vi "save_scope_config.vi"(0 "Current VI's Path":path=path "" caption="start path", 2 "Save File Type":u16(ring) items=["Automatic Save", "Custom File"], 7 "Controls cluster":T4 {"C1 vertical coupling / V" items=["AC", "DC", "Ground"]; "C2 vertical coupling / V" items=["AC", "DC", "Ground"]; "Trigger slope" items=["Positive", "Negative"]}, 11 "error in":errorcluster) -> (8 "Controls cluster out":T4 {"C1 vertical coupling / V" items=["AC", "DC", "Ground"]; "C2 vertical coupling / V" items=["AC", "DC", "Ground"]; "Trigger slope" items=["Positive", "Negative"]}, 15 "error out":errorcluster)   [LabVIEW 2023]
uses:
  <instrlib>/niScope/Controls/niScope vertical coupling.ctl
  <instrlib>/niScope/Controls/niScope trigger source.ctl
  <instrlib>/niScope/Controls/niScope trigger slope.ctl
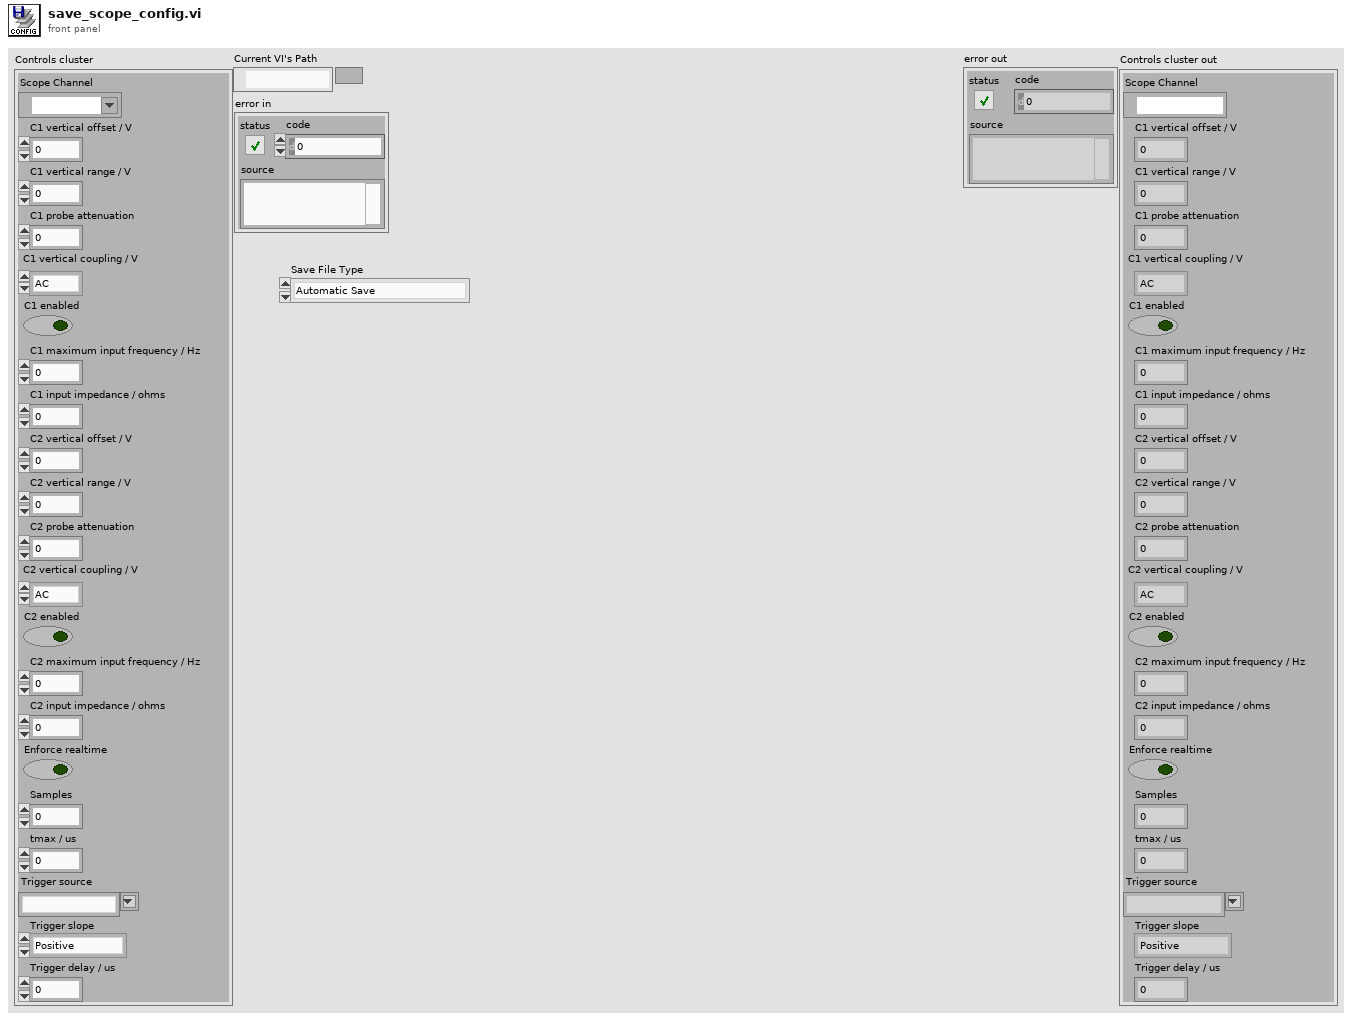
[diagram p1: front panel]
types:
  T1 = typedef "niScope vertical coupling.ctl" = i32
  T2 = typedef "niScope trigger source.ctl" = string
  T3 = typedef "niScope trigger slope.ctl" = i32
  T4 = cluster{"Scope Channel":refnum<k15>, "C1 vertical offset / V":dbl, "C1 vertical range / V":dbl, "C1 probe attenuation":dbl, "C1 vertical coupling / V":T1, "C1 enabled":bool, "C1 maximum input frequency / Hz":dbl, "C1 input impedance / ohms":u32, "C2 vertical offset / V":dbl, "C2 vertical range / V":dbl, "C2 probe attenuation":dbl, "C2 vertical coupling / V":T1, "C2 enabled":bool, "C2 maximum input frequency / Hz":dbl, "C2 input impedance / ohms":u32, "Enforce realtime":bool, "Samples":i64, "tmax / us ":dbl, "Trigger source":T2, "Trigger slope":T3, "Trigger delay / us":dbl}
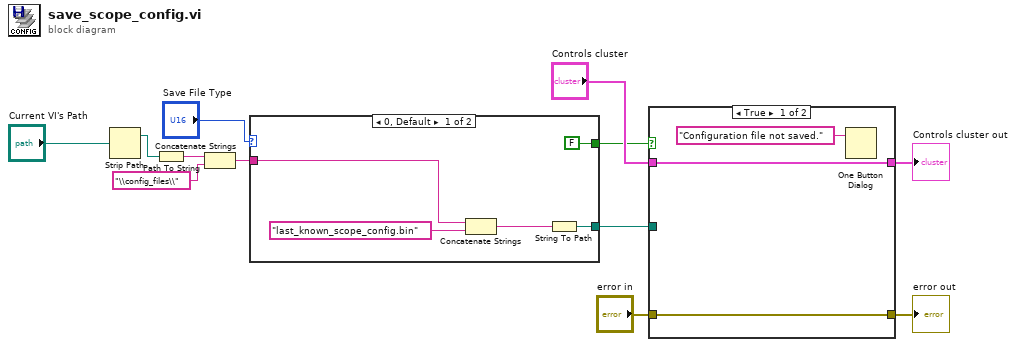
[diagram p0: block diagram]
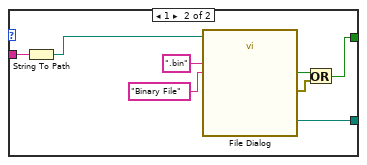
[diagram p2: hidden frame]
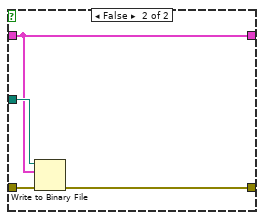
[diagram p3: hidden frame]
diagram:
  n1 = Strip Path(path="Current VI's Path") -> (stripped path=w5:path)  [unwired: 1 out]
  n2 = Path To String(path=w5) -> (string=w4:string)
  n3 = Concatenate Strings(w4, "\\config_files\\" ("string")) -> (w2:string)
  n4 = case shown="0, Default" "Save File Type" {
    tunnel: [FALSE w21] -> w7
    tunnel: [w14 w20] -> w6
    tunnel: w2 -> [w17 w19]
    frame 0, Default {
      n5 = Concatenate Strings(w17, "last_known_scope_config.bin" ("string")) -> (w15:string)
      n6 = String To Path(string=w15) -> (path=w14:path)
    }
    frame 1 {
      n7 = String To Path(string=w19) -> (path=w18:path)
      n8 = call "File Dialog"("start path"=w18, "pattern (all files)"=".bin", "pattern label"="Binary File") -> ("selected path"=w20:path, "cancelled"=w25:bool, "error out"=w24:errorcluster)  [unwired: 9 in, 1 out]
      n9 = Or(x=w25, y=w24) -> (x .or. y?=w21:bool)
    }
  }
  n10 = case shown="True" w7 {
    tunnel: "Controls cluster" -> [w27 w29]
    tunnel: "error in" -> [w28 w32]
    tunnel: [w28 w31] -> w10
    tunnel: w6 -> [_ w30]
    tunnel: [w27 w29] -> w9
    frame True {
      n11 = One Button Dialog(message="Configuration file not saved.") -> ()  [unwired: 1 in, 1 out]
    }
    frame False {
      n12 = Write to Binary File(file (use dialog)=w30, data=w29, error in=w32) -> (error out=w31:errorcluster)  [unwired: 3 in, 2 out]
    }
  }
  "error out" <- w10
  "Controls cluster out" <- w9
